vi "Generate Single Tone Waveform.vi"(8 "error in":errorcluster, 9 "DAQmx product type":string, 10 "Measurement Configuration":T1={"Band start"=20.0, "Band stop"=20000.0, "Weighting filter"="Linear", "Amplitude"=1.0, "Frequency"=1000.0, "Full scale range"=3.16, "Analog source resource name"="", "Protocol capture resource name"="", "Channel name"="0L", "Data line"=0, "Sample rate"=12288000.0, "Measurement duration"=19200.0, "Channel"=0, "Frame sync edge for channel 0"=0, "Channel count per frame"=0, "Channel length"=32, "Bit depth"=24, "Channel 0 offset"=1, "Endianness"=0, "Data justification"=0, "Frame length"=64, "Frame sync pulse width"=32, "Bit clock edge sync"=1} {"Data line" format="%#.0f"}, 11 "DSG task in":refnum<k21>) -> (0 "error out":errorcluster, 3 "DSG task out":refnum<k21>)   [LabVIEW 2021, in "audio_adc_acMeasurement.lvlib"]
uses:
  audio_adc_acMeasurement.lvlib
  <vilib>/addons/_NISVFA/_Generation/Signal Generation/SV Signal/sv_System Timing Model.ctl
  <vilib>/addons/_NISVFA/_Generation/Signal Generation/SV Signal/SV Signal.lvclass
  <resource>/objmgr/daqmx.rc
  <vilib>/addons/_NISVFA/_Generation/Signal Generation/SV Sinusoid/Configure Sine.vi
  <vilib>/addons/_NISVFA/_Generation/Signal Generation/SV Sinusoid/SV Sinusoid.lvclass
  <vilib>/DAQmx/write.llb/DAQmx Write (Analog 1D Wfm NChan NSamp).vi
  Measurement Configuration.ctl
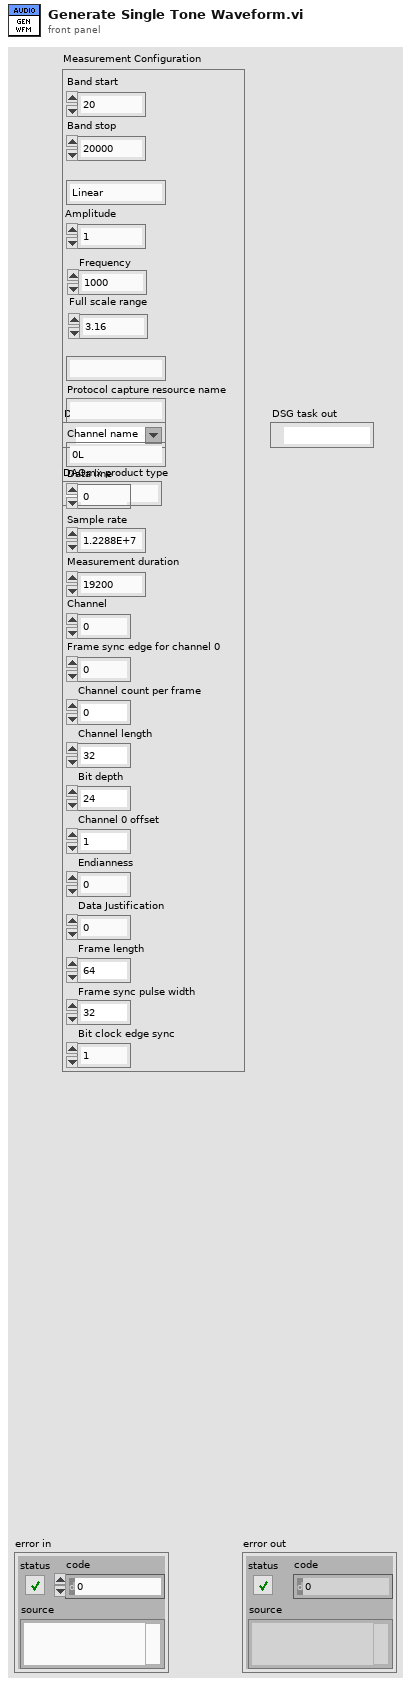
[diagram p1: front panel]
types:
  T1 = typedef "audio_adc_acMeasurement.lvlib/Measurement Configuration.ctl" = cluster{"Band start":dbl, "Band stop":dbl, "Weighting filter":string, "Amplitude":dbl, "Frequency":dbl, "Full scale range":dbl, "Analog source resource name":string, "Protocol capture resource name":string, "Channel name":string, "Data line":u16, "Sample rate":dbl, "Measurement duration":dbl, "Channel":u32, "Frame sync edge for channel 0":u32, "Channel count per frame":u32, "Channel length":u32, "Bit depth":u32, "Channel 0 offset":u32, "Endianness":u32, "Data justification":u32, "Frame length":u32, "Frame sync pulse width":u32, "Bit clock edge sync":u32}
  T2 = cluster{"profile":enum16{"Linear", "Half cosine"}, "durations [s]":cluster{"ramp-up":dbl, "transition":dbl, "ramp-down":dbl}}
  T3 = typedef "SV Signal.lvclass/sv_System Timing Model.ctl" = i64
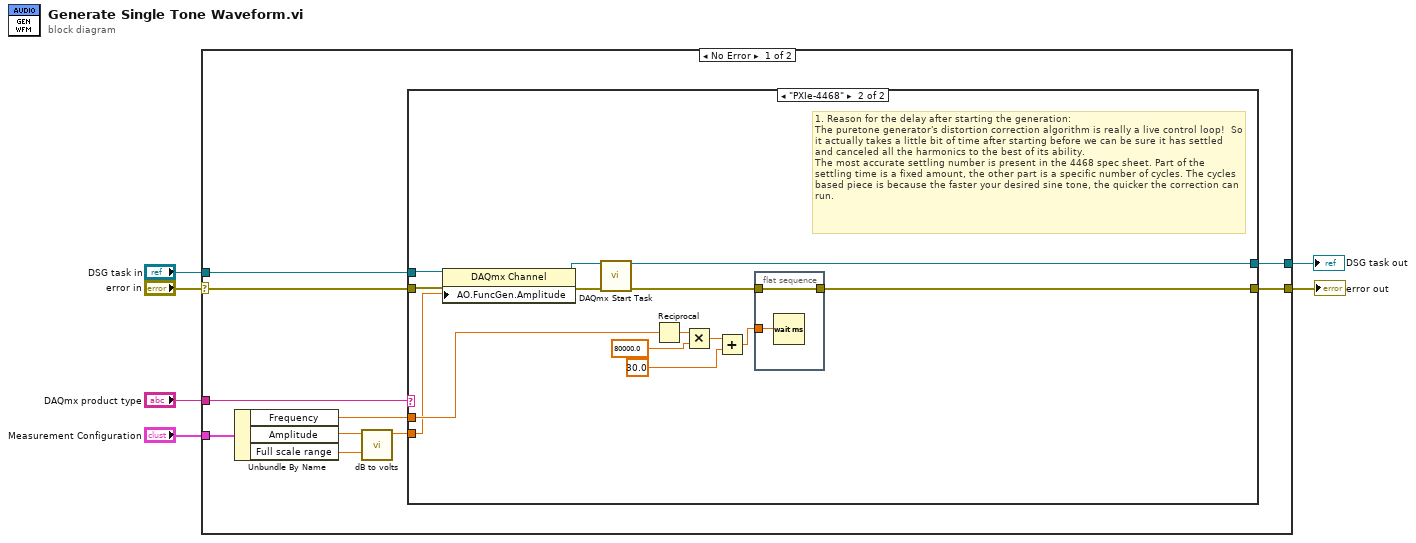
[diagram p0: block diagram]
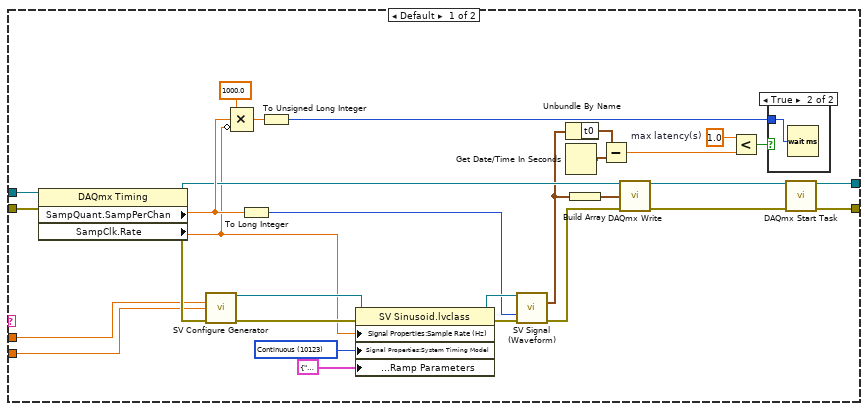
[diagram p2: hidden frame]
diagram:
  n1 = case shown="No Error" "error in" {
    selector: "error in" -> [w13 w64]
    tunnel: [w16 w65] -> w6
    tunnel: "DSG task in" -> [w15 w65]
    tunnel: [w14 w64] -> w4
    tunnel: "Measurement Configuration" -> [w12 _]
    tunnel: "DAQmx product type" -> [w8 _]
    frame No Error {
      n2 = Unbundle By Name(w12) -> ("Frequency"=w11:dbl, "Amplitude"=w10:dbl, "Full scale range"=w7:dbl)
      n3 = call "dB to volts.vi"("Full scale range"=w7, "Voltage(dB)"=w10) -> ("Voltage(volts)"=w9:dbl)  [unwired: 9 in]
      n4 = case shown="\"PXIe-4468\"" w8 {
        tunnel: [w19 w61] -> w14
        tunnel: w15 -> [w33 w52]
        tunnel: w13 -> [w32 w50]
        tunnel: [w20 w54] -> w16
        tunnel: w11 -> [w18 w53]
        tunnel: w9 -> [w17 w48]
        frame Default {
          w38 = 1.0  # max latency(s)
          w44 = T3 10123 items=["Finite"=10178, "-"=-1, "Continuous"=10123, "-"=-2, "Settled"=110123, "Averaged"=210123, "Discrete Sweep"=310123, "Continuous Sweep"=410123] ("System Timing Model")
          n5 = property class="DAQmx Timing"(reference=w33, error in=w32) -> (reference out=w39:refnum<k21>, error out=w22:errorcluster, "SampQuant.SampPerChan"=w41:dbl, "SampClk.Rate"=w21:dbl)
          n6 = call-poly <vilib>:"SV Configure Generator.vi"("frequency (Hz)"=w18, "amplitude"=w17, "error in (no error)"=w22) -> ("signal configuration"=w45:refnum<class "SV Sinusoid.lvclass">, "error out"=w46:errorcluster)  [unwired: 11 in]
          n7 = Compound Arithmetic op=MULTIPLY(1000.0 ("value"), w41, invert w21) -> (w37:dbl)
          n8 = To Long Integer(number=w41) -> (32bit integer=w40:i32)
          n9 = To Unsigned Long Integer(number=w37) -> (unsigned 32bit integer=w35:u32)
          n10 = property class="SV Sinusoid.lvclass"(reference=w45, error in=w46, "Signal Properties:Sample Rate (Hz)"=w21, "Signal Properties:System Timing Model"=w44, "Signal Properties:Ramps:Ramp Parameters"=T2 {"profile"=enum."Linear", "durations [s]"={"ramp-up"=0.0, "transition"=0.0, "ramp-down"=0.01}} ("Ramp Parameters:All Elements")) -> (reference out=w43:refnum<class "SV Sinusoid.lvclass">, error out=w42:errorcluster)
          n11 = call-dynamic "SV Signal (Waveform).vi"("signal configuration"=w43, "samples"=w40, "error in (no error)"=w42) -> ("output waveform"=w29:waveform(dbl), "error out"=w30:errorcluster)  [unwired: 7 in, 4 out]
          n12 = Unbundle By Name(w29) -> ("t0"=w28:timestamp)
          n13 = Get Date/Time In Seconds() -> (seconds since 1Jan1904=w27:timestamp)
          n14 = Build Array(w29) -> (w31:waveform(dbl)[])
          n15 = Subtract(x=w28, y=w27) -> (x-y=w26:dbl)
          n16 = call-poly <vilib>:"DAQmx Write.vi"("task/channels in"=w39, "data"=w31, "error in"=w30) -> ("task out"=w24:refnum<k21>, "error out"=w23:errorcluster)  [unwired: 10 in, 1 out]
          n17 = Less?(x=w38, y=w26) -> (x < y?=w25:bool)
          n18 = case shown="True" w25 {
            tunnel: w35 -> [_ w47]
            frame False {
            }
            frame True {
              n19 = Wait (ms)(milliseconds to wait=w47) -> ()  [unwired: 1 out]
            }
          }
          n20 = call <vilib>:"DAQmx Start Task.vi"("task/channels in"=w24, "error in"=w23) -> ("task out"=w20:refnum<k21>, "error out"=w19:errorcluster)  [unwired: 12 in]
        }
        frame "PXIe-4468" {
          # "1. Reason for the delay after starting the generation: \nThe puretone generator's distortion correction algorithm is really a live control loop!  So it actually takes a little bit of time after starting before we can be sure it has settled and canceled all the harmonics to the best of its ability. \nThe most accurate settling number is present in the 4468 spec sheet. Part of the settling time is a fixed amount, the other part is a specific number of cycles. The cycles based piece is because the faster your desired sine tone, the quicker the correction can run."
          n21 = property class="DAQmx Channel"(reference=w52, error in=w50, "AO.FuncGen.Amplitude"=w48) -> (reference out=w51:refnum<k21>, error out=w49:errorcluster)
          n22 = call <vilib>:"DAQmx Start Task.vi"("task/channels in"=w51, "error in"=w49) -> ("task out"=w54:refnum<k21>, "error out"=w60:errorcluster)  [unwired: 12 in]
          n23 = Reciprocal(x=w53) -> (1/x=w59:dbl)
          n24 = Multiply(x=w59, y=80000.0) -> (x*y=w57:dbl)
          n25 = Add(x=w57, y=30.0) -> (x+y=w55:dbl)
          n26 = flat-sequence {
            tunnel: [w63] -> w61
            tunnel: w60 -> [w63]
            tunnel: w55 -> [w62]
            frame #0 {
              n27 = Wait (ms)(milliseconds to wait=w62) -> ()  [unwired: 1 out]
            }
          }
        }
      }
    }
    frame Error {
    }
  }
  "DSG task out" <- w6
  "error out" <- w4
